vi "Crop Frame.vi"(7 "Cropped Frame":T1, 8 "error in (no error)":errorcluster, 9 "Frame":T1, 10 "Crop ROI":i32[](array[numeric]), 11 "Mask":T1) -> (0 "error out":errorcluster, 3 "Cropped Frame Out":T1)   [LabVIEW 2017]
uses:
  <vilib>/vision/Image Controls.llb/IMAQ Image.ctl
  <vilib>/vision/NI_Vision_Development_Module.lvlib
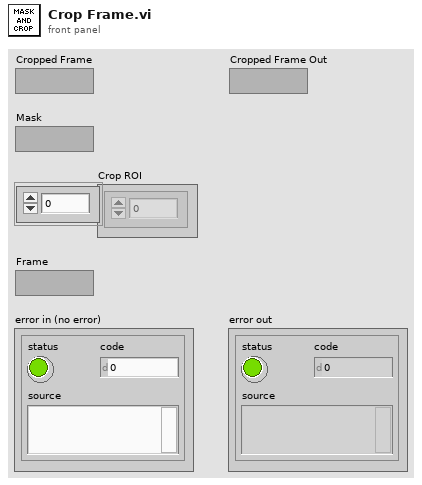
[diagram p1: front panel]
types:
  T1 = typedef "IMAQ Image.ctl" = refnum<image>
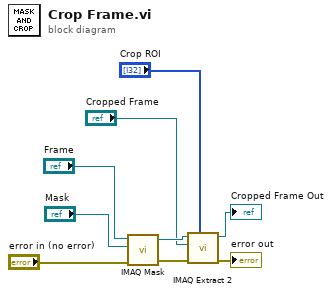
[diagram p0: block diagram]
diagram:
  n1 = call "IMAQ Mask"("error in (no error)"="error in (no error)", "Image Mask"="Mask", "Image Src"="Frame") -> ("error out"=w6:errorcluster, "Image Dst Out"=w9:T1)  [unwired: 2 in]
  n2 = call "IMAQ Extract 2"("Optional Rectangle"="Crop ROI", "error in (no error)"=w6, "Image Dst"="Cropped Frame", "Image Src"=w9) -> ("error out"=→"error out":errorcluster, "Image Dst Out"=→"Cropped Frame Out":T1)  [unwired: 6 in]
